vi "ziExample-InitializeParameters.vi"() -> ()   [LabVIEW 2009]
doc: "Control a Zurich Instruments device via a LabOne Labview API.\nExample from the Getting Started guide: An array of parameters is element-wise set. The procedure is a useful building block that ensures to always measure with the same settings.\n\n© Zurich Instruments AG, www.zhinst.com"
uses:
  <instrlib>/Zurich Instruments LabOne/Public/Configure/ziGetValueDouble.vi
  <instrlib>/Zurich Instruments LabOne/Public/Configure/ziSetValueDouble.vi
  <instrlib>/Zurich Instruments LabOne/Public/Configure/ziSetValueDoubleArray.vi
  <instrlib>/Zurich Instruments LabOne/Zurich Instruments LabOne.lvlib
panel:
  out "Error Out":errorcluster
  in  "setNODE":string="oscs/0/freq"
  in  "setVALUE":dbl=123456.0
  out "getVALUE":dbl
  in  "Address":string="DEV"
  out "Selected Device":string
  # "ziExample-InitializeParameters.vi\nRequirements: HF2, UHFLI or MFLI see block diagram for VI description"
  # "Tested Devices:\n- HF2LI, HF2IS\n- UHFLI\n- MFLI"
  # "SEE DIAGRAM\nFOR further INFOs."
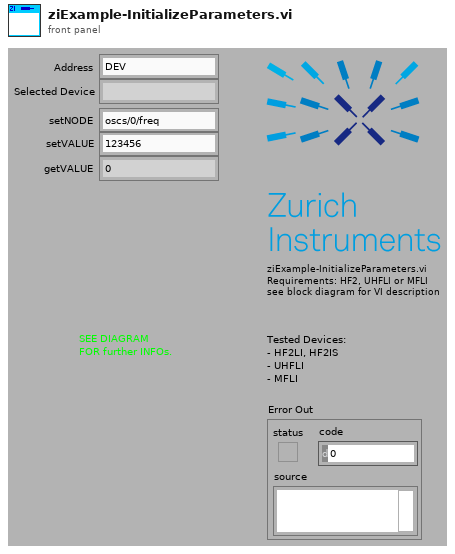
[diagram p1: front panel]
types:
  T1 = typedef "Zurich Instruments LabOne.lvlib/ziTypeHandle.ctl" = cluster{"handleValid":bool, "Conn":u64, "Path Prefix":string, "Handle":u64, "Connected":bool, "Clockbase(s)":dbl}
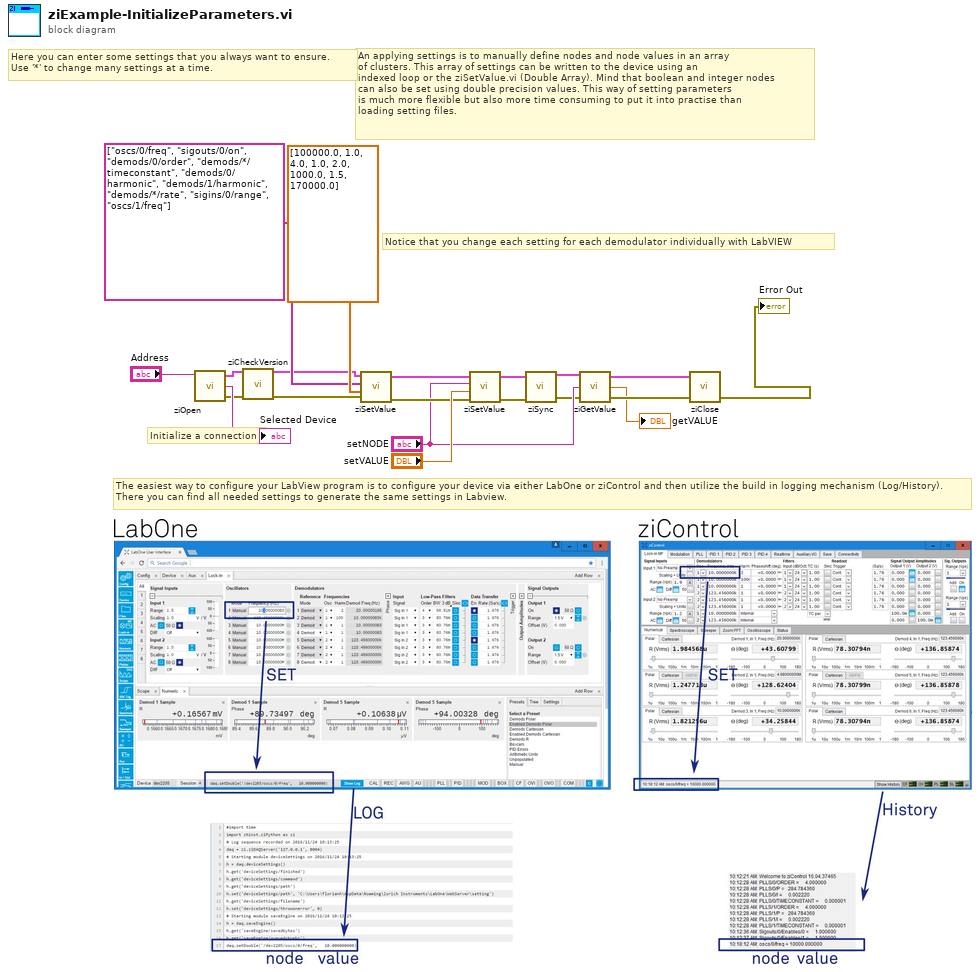
[diagram p0: block diagram]
diagram:
  # "The easiest way to configure your LabView program is to configure your device via either LabOne or ziControl and then utilize the build in logging mechanism (Log/History). There you can find all needed settings to generate the same settings in Labview."
  # "Initialize a connection"
  # "An applying settings is to manually define nodes and node values in an array \nof clusters. This array of settings can be written to the device using an \nindexed loop or the ziSetValue.vi (Double Array). Mind that boolean and integer nodes \ncan also be set using double precision values. This way of setting parameters \nis much more flexible but also more time consuming to put it into practise than \nloading setting files."
  # "Notice that you change each setting for each demodulator individually with LabVIEW"
  # "Here you can enter some settings that you always want to ensure.\nUse '*' to change many settings at a time."
  n1 = call <instrlib>:"ziOpen.vi"("Address"="Address") -> ("Error Out"=w7:errorcluster, "Selected Device"=→"Selected Device":string, "HandleOut"=w8:T1)  [unwired: 1 in, 2 out]
  n2 = call <instrlib>:"ziCheckVersion.vi"("Handle In"=w8, "Error In"=w7) -> ("Handle Out"=w5:T1, "Error Out"=w6:errorcluster)  [unwired: 11 in, 1 out]
  n3 = call-poly <instrlib>:"ziSetValue.vi"("Error In"=w6, "Values"=dbl[] [100000.0, 1.0, 4.0, 1.0, 2.0, 1000.0, 1.5, 170000.0], "Paths"=string[] ["oscs/0/freq", "sigouts/0/on", "demods/0/order", "demods/*/timeconstant", "demods/0/harmonic", "demods/1/harmonic", "demods/*/rate", "sigins/0/range", "oscs/1/freq"], "Handle In"=w5) -> ("Error Out"=w14:errorcluster, "Handle Out"=w15:T1)  [unwired: 1 in]
  n4 = call-poly <instrlib>:"ziSetValue.vi"("Error In"=w14, "Value"="setVALUE", "Path"="setNODE", "Handle In"=w15) -> ("Error Out"=w1:errorcluster, "Handle Out"=w4:T1)  [unwired: 1 in]
  n5 = call <instrlib>:"ziSync.vi"("Handle In"=w4, "Error In"=w1) -> ("Handle Out"=w3:T1, "Error Out"=w2:errorcluster)  [unwired: 12 in]
  n6 = call-poly <instrlib>:"ziGetValue.vi"("error in"=w2, "Path"="setNODE", "Handle in"=w3) -> ("error out"=w11:errorcluster, "Value"=→"getVALUE":dbl, "Handle out"=w12:T1)
  n7 = call <instrlib>:"ziClose.vi"("Error In"=w11, "Handle In"=w12) -> ("Error Out"=→"Error Out":errorcluster)  [unwired: 2 in, 1 out]
